vi "Remove Log File.vi"(8 "error in":errorcluster, 11 "log file":T1 format="%.0x") -> (0 "error out":errorcluster)   [LabVIEW 2027, in "Embedded Data Logger Scripting.lvlib"]
uses:
  Embedded Data Logger Scripting.lvlib
  <vilib>/NI VeriStand/Custom Device API/Custom Device Item Ref.ctl
  <vilib>/NI VeriStand/Custom Device API/Custom Device API.lvlib
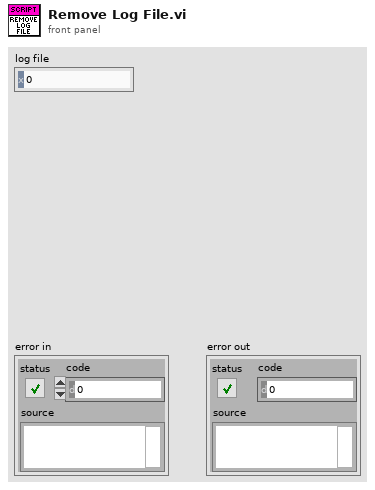
[diagram p1: front panel]
types:
  T1 = typedef "Custom Device API.lvlib/Custom Device Item Ref.ctl" = u64
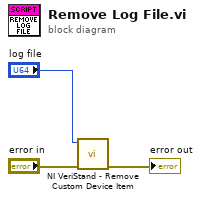
[diagram p0: block diagram]
diagram:
  n1 = call <vilib>:"NI VeriStand - Remove Custom Device Item.vi"("error in (no error)"="error in", "Item Ref in"="log file") -> ("error out"=→"error out":errorcluster)  [unwired: 8 in, 1 out]
